vi "Gyro Get Mode.vi"(11 "I2CDevRef":T2 {"Device Address" format="%.0x"}) -> (2 "DPS Mode":T1, 3 "I2CDevRef Out":T2 {"Device Address" format="%.0x"})   [LabVIEW 2013]
uses:
  <vilib>/Rock Robotics/WPI/I2C/WPI_I2CDevRef.ctl
  <vilib>/Rock Robotics/SystemInterfaces/Typedef/FPGA_TypedefDigitalModule.ctl
  DPS Mode.ctl
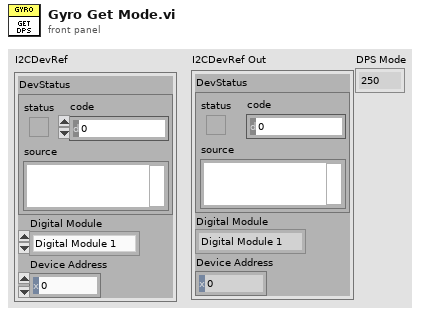
[diagram p1: front panel]
types:
  T1 = typedef "DPS Mode.ctl" = enum16{"250", "500", "2000"}
  T2 = typedef "WPI_I2CDevRef.ctl" = cluster{"DevStatus":errorcluster, "Digital Module":T3, "Device Address":u8}
  T3 = typedef "FPGA_TypedefDigitalModule.ctl" = enum16{"Digital Module 1", "Digital Module 2"}
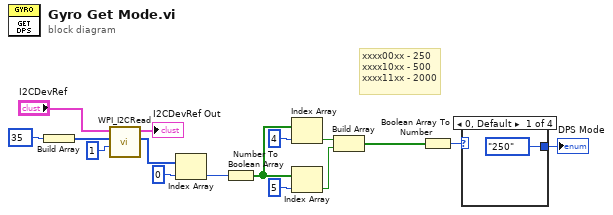
[diagram p0: block diagram]
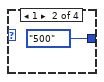
[diagram p2: hidden frame]
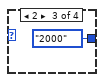
[diagram p3: hidden frame]
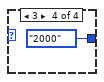
[diagram p4: hidden frame]
diagram:
  # "xxxx00xx - 250\nxxxx10xx - 500\nxxxx11xx - 2000"
  n1 = Build Array(u8 35 ("Data To Send")) -> (w10:u8[])
  n2 = call <vilib>:"WPI_I2CRead.vi"("I2CBytesToRead"=u8 1, "I2CRegister"=w10, "I2CDevRef"="I2CDevRef") -> ("Data Out"=w14:u8[], "I2CDevRef"=→"I2CDevRef Out":T2)  [unwired: 6 in, 1 out]
  n3 = Index Array(array=w14, index=0) -> (element=w12:u8)
  n4 = Number To Boolean Array(number=w12) -> (Boolean array=w6:bool[])
  n5 = Index Array(array=w6, index=4) -> (element=w5:bool)
  n6 = Index Array(array=w6, index=5) -> (element=w4:bool)
  n7 = Build Array(w5, w4) -> (w3:bool[])
  n8 = Boolean Array To Number(Boolean array=w3) -> (number=w2:u32)
  n9 = case shown="0, Default" w2 {
    tunnel: [DPS_Mode."250" ("DPS Mode") DPS_Mode."500" ("DPS Mode") DPS_Mode."2000" ("DPS Mode") DPS_Mode."2000" ("DPS Mode")] -> w1
    frame 0, Default {
    }
    frame 1 {
    }
    frame 2 {
    }
    frame 3 {
    }
  }
  "DPS Mode" <- w1
